vi "Set_Tunnel_Speed_server.vi"(3 "Tunnel Velocity m/s":dbl min=0.0 max=50.0 format="%.2f", 4 "Rig Name":string, 5 "Mode":T1, 6 "Client Name":string="G3_3 HD") -> (0 "Error String":string, 1 "Settling Time (s)":dbl format="%.2f", 2 "Valid Client":bool)   [LabVIEW 2010]
uses:
  ADAM Client/Sub VIs/ADAM Controls/Tunnel_speed_mode.ctl
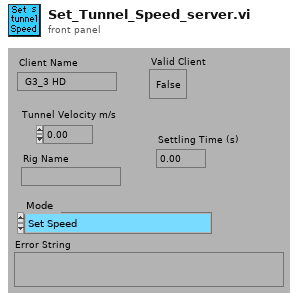
[diagram p1: front panel]
types:
  T1 = typedef "Tunnel_speed_mode.ctl" = enum16{"Set Speed", "Set Speed then wait", "Is tunnel speed allowable?"}
  T2 = typedef "Ch_description_ADAM.ctl" = cluster{"Ch Name":string, "Type":T3, "Function":T4, "Ch State":T5, "Calibration type":T6, "A":dbl, "B":dbl, "C":dbl, "D":dbl, "Comments":string, "Address":T7, "String":string, "Duty":u16}
  T3 = typedef "Module_type_ADAM.ctl" = enum16{"4011", "4012", "4013", "4014", "4016", "4017", "4018", "4021", "4050", "4052", "4053", "4060", "4080", "5000", "5017", "5018", "5024", "5051", "5056", "5060", "6060", "Tracker", "WEST", "GILL", "JEM", "VICI", "Vaisala", "DRUCK", "Run VI Named:", "IR2100", "PPT", "Comparator", "VIRTUAL", "Hold Value", "Read A", "Read Ch", "Coded", "Client Info", "Web Client", "X10", "Test"}
  T4 = typedef "Function_ADAM.ctl" = enum16{"Analogue Input", "Digital Input", "Event counter", "Event rate", "Analogue Output", "Digital Output", "Relay Output"}
  T5 = typedef "Channel_State.ctl" = enum16{"On", "Off", "Always On", "Always Off"}
  T6 = typedef "Calib_type_ADAM.ctl" = enum16{"Raw", "Bx + A", "Cx^2 + Bx + A", "Dx^3 + Cx^2 + Bx + A", "In Band", "Hi-Tec Q", "Hi-Tec M_dot", "Text"}
  T7 = typedef "Address.ctl" = cluster{"Main":i32, "Ch.":i32, "Sub":i32, "Port Name":string}
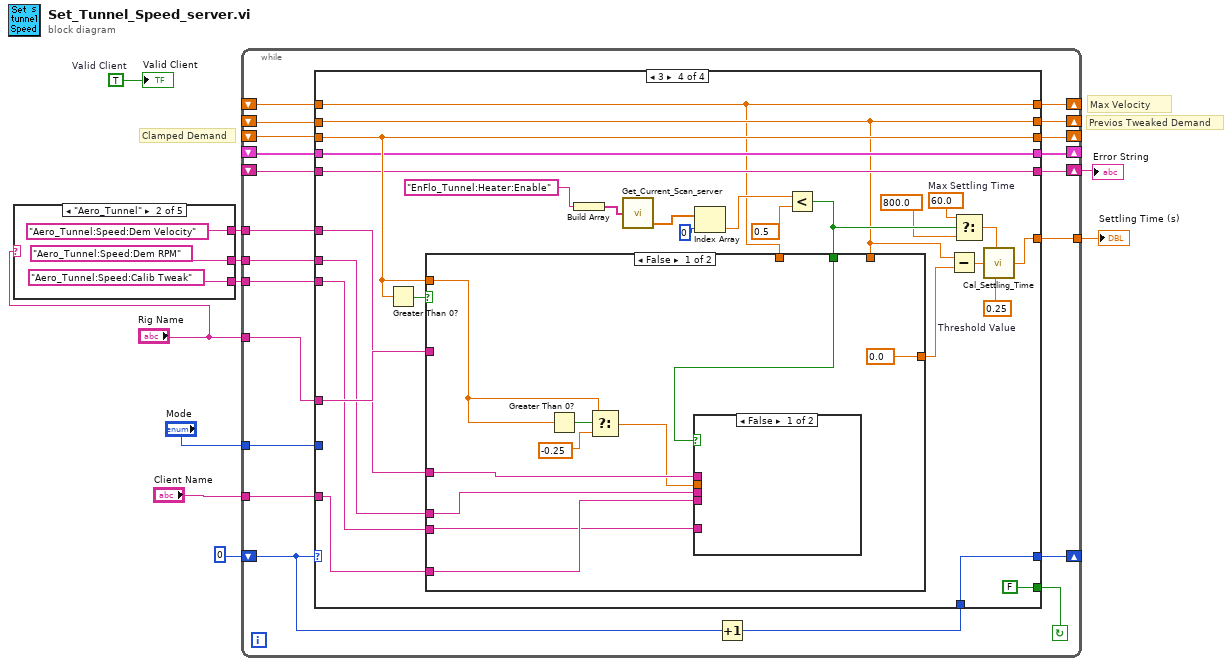
[diagram p0: block diagram]
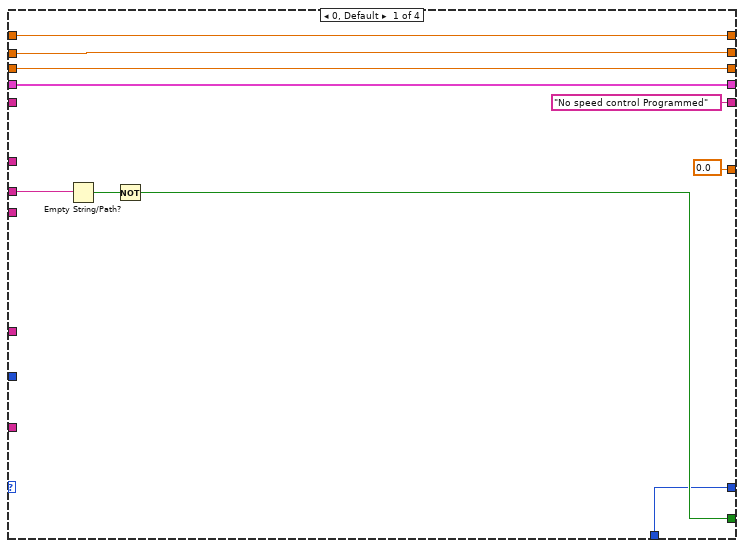
[diagram p2: hidden frame]
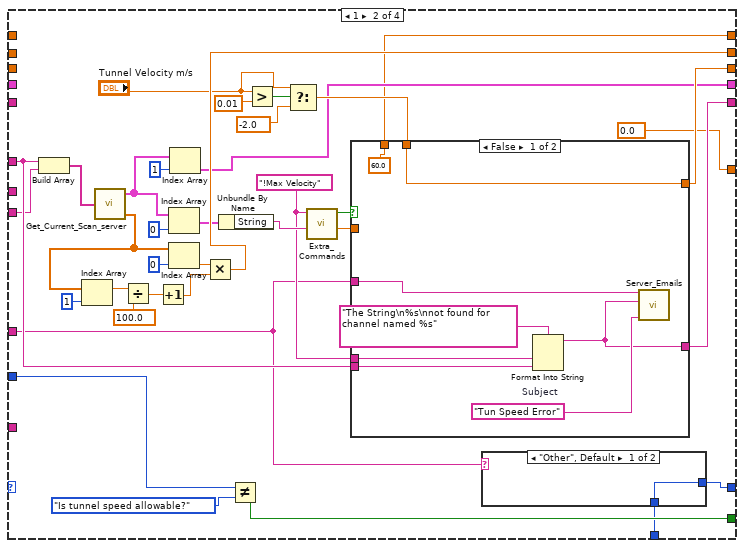
[diagram p3: hidden frame]
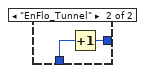
[diagram p4: hidden frame]
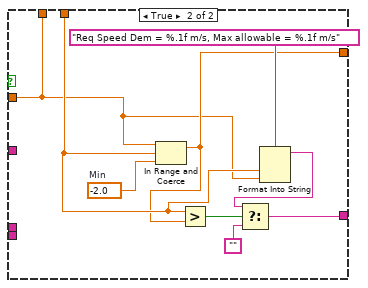
[diagram p5: hidden frame]
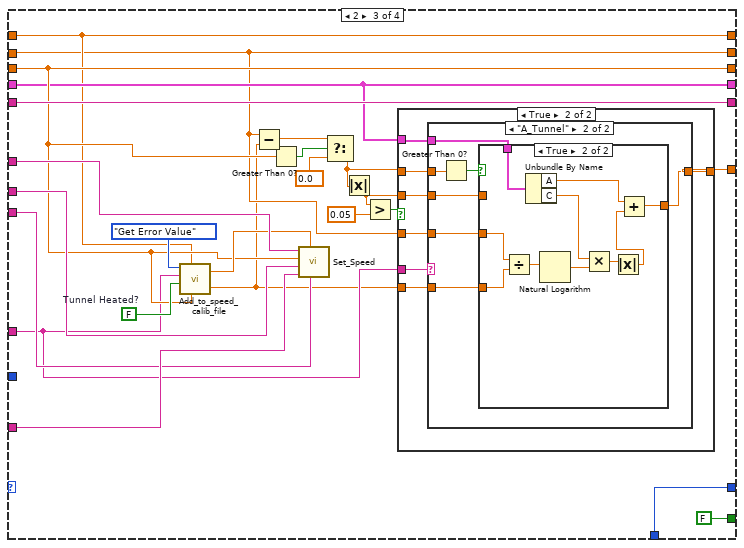
[diagram p6: hidden frame]
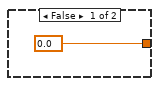
[diagram p7: hidden frame]
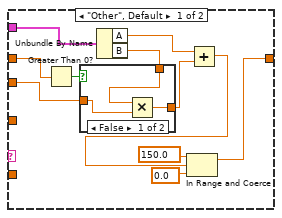
[diagram p8: hidden frame]
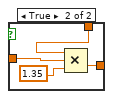
[diagram p9: hidden frame]
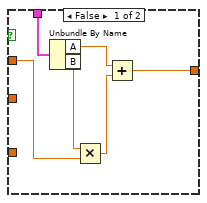
[diagram p10: hidden frame]
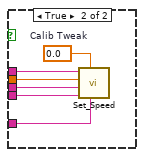
[diagram p11: hidden frame]
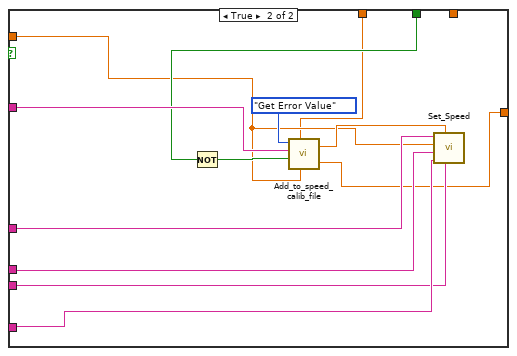
[diagram p12: hidden frame]
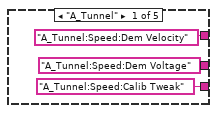
[diagram p13: hidden frame]
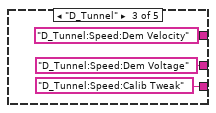
[diagram p14: hidden frame]
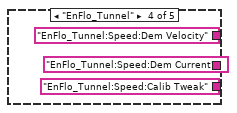
[diagram p15: hidden frame]
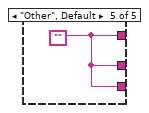
[diagram p16: hidden frame]
diagram:
  w10 = TRUE  # Valid Client
  # "Max Velocity"
  # "Previos Tweaked Demand"
  # "Clamped Demand"
  n1 = case shown="\"Aero_Tunnel\"" "Rig Name" {
    tunnel: ["A_Tunnel:Speed:Dem Velocity" "Aero_Tunnel:Speed:Dem Velocity" "D_Tunnel:Speed:Dem Velocity" "EnFlo_Tunnel:Speed:Dem Velocity" w23] -> w6
    tunnel: ["A_Tunnel:Speed:Dem Voltage" "Aero_Tunnel:Speed:Dem RPM" "D_Tunnel:Speed:Dem Voltage" "EnFlo_Tunnel:Speed:Dem Current" w23] -> w3
    tunnel: ["A_Tunnel:Speed:Calib Tweak" "Aero_Tunnel:Speed:Calib Tweak" "D_Tunnel:Speed:Calib Tweak" "EnFlo_Tunnel:Speed:Calib Tweak" w23] -> w1
    frame "A_Tunnel" {
    }
    frame "Aero_Tunnel" {
    }
    frame "D_Tunnel" {
    }
    frame "EnFlo_Tunnel" {
    }
    frame "Other", Default {
      w23 = ""
    }
  }
  n2 = while {
    shift-left: _ -> [w26]
    shift-right: [w27] -> _
    tunnel: w1 -> [w28]
    shift-left: _ -> [w30]
    shift-right: [w29] -> _
    tunnel: [w31] -> w2
    tunnel: w3 -> [w33]
    shift-left: _ -> [w32]
    shift-right: [w36] -> w5
    shift-left: _ -> [w34]
    shift-right: [w37] -> _
    tunnel: w6 -> [w38]
    shift-left: 0 -> [w41]
    shift-right: [w40] -> _
    tunnel: "Client Name" -> [w43]
    tunnel: "Mode" -> [w44]
    tunnel: "Rig Name" -> [w42]
    shift-right: [w25] -> _
    shift-left: _ -> [w24]
    stop <- w35 continue-if-true
    n3 = Increment(x=w41) -> (x+1=w39:i32)
    n4 = case shown="3" w41 {
      tunnel: w34 -> [w50 _ w122 w199]
      tunnel: w44 -> [_ w80 _ _]
      tunnel: ["No speed control Programmed" w82 w129 w195] -> w36
      tunnel: w43 -> [_ _ w134 w209]
      tunnel: w42 -> [_ w71 w113 w208]
      tunnel: [w51 w74 w132 w200] -> w40
      tunnel: w39 -> [w51 w75 w132 w200]
      tunnel: w38 -> [_ w85 w131 w203]
      tunnel: [w50 w83 w122 w199] -> w37
      tunnel: [w52 w79 FALSE FALSE] -> w35
      tunnel: w33 -> [w54 _ w130 w202]
      tunnel: w32 -> [_ _ w129 w195]
      tunnel: [0.0 ("Settling Time") 0.0 ("Settling Time") w119 w197] -> w31
      tunnel: w30 -> [w48 _ w112 w187]
      tunnel: [w48 w62 w112 w187] -> w29
      tunnel: w28 -> [_ w70 w124 w190]
      tunnel: [w46 w56 w118 w188] -> w27
      tunnel: w26 -> [w46 _ w118 w188]
      tunnel: [w45 w55 w115 w184] -> w25
      tunnel: w24 -> [w45 _ w115 w184]
      frame 0, Default {
        n5 = Empty String/Path?(string/path=w54) -> (empty?=w53:bool)
        n6 = Not(x=w53) -> (.not. x?=w52:bool)
      }
      frame 1 {
        w86 = "!Max Velocity" ("Command")
        n7 = Build Array(w85, w70) -> (w90:string[])
        n8 = call "Get_Current_Scan_server.vi"("Desired Channels"=w90) -> ("Ch Description Array"=w57:T2[], "Numerical Values"=w68:dbl[])  [unwired: 1 out]
        n9 = Index Array(array=w68, index=1 ("Index")) -> (element=w67:dbl)
        n10 = Divide(x=w67, y=100.0) -> (x/y=w65:dbl)
        n11 = Increment(x=w65) -> (x+1=w63:dbl)
        n12 = Index Array(array=w57, index=0 ("Index")) -> (element=w59:T2)
        n13 = Index Array(array=w68, index=0 ("Index")) -> (element=w64:dbl)
        n14 = Index Array(array=w57, index=1 ("Index")) -> (element=w56:T2)
        n15 = Multiply(x=w64, y=w63) -> (x*y=w62:dbl)
        n16 = Unbundle By Name(w59) -> ("String"=w88:string)
        n17 = Not Equal?(x=w80, y=Tunnel_speed_mode."Is tunnel speed allowable?" ("Mode")) -> (x != y?=w79:bool)
        n18 = Greater?(x="Tunnel Velocity m/s", y=0.01) -> (0:w78:bool)
        n19 = Select(t="Tunnel Velocity m/s", s=w78, f=-2.0 ("t")) -> (s? t:f=w76:dbl)
        n20 = call "Extra_Commands.vi"("String to Search"=w88, "Command"=w86) -> ("Numeric Value"=w84:dbl, "Command Found"=w87:bool)  [unwired: 1 in, 3 out]
        n21 = case shown="False" w87 {
          tunnel: w71 -> [w95 _]
          tunnel: w86 -> [w100 _]
          tunnel: w85 -> [w99 _]
          tunnel: w84 -> [_ w102]
          tunnel: w76 -> [w97 w104]
          tunnel: [w97 w103] -> w83
          tunnel: [w96 w106] -> w82
          tunnel: [60.0 ("Numeric Value") w102] -> w55
          frame False {
            w101 = "Tun Speed Error"  # Subject
            n22 = Format Into String(format string="The String\n%s\nnot found for channel named %s" ("Format String"), w100, w99) -> (resulting string=w96:string)  [unwired: 2 in, 1 out]
            n23 = call "Server_Emails.vi"("Client Name Contains"=w95, "Message"=w96, "Subject"=w101) -> ()  [unwired: 2 in, 3 out]
          }
          frame True {
            w110 = -2.0  # Min
            n24 = In Range and Coerce(upper limit=w102, x=w104, lower limit=w110) -> (coerced(x)=w103:dbl)  [unwired: 1 out]
            n25 = Greater?(x=w104, y=w103) -> (0:w105:bool)
            n26 = Format Into String(format string="Req Speed Dem = %.1f m/s, Max allowable = %.1f m/s", w104, w102) -> (resulting string=w108:string)  [unwired: 2 in, 1 out]
            n27 = Select(t=w108, s=w105, f="") -> (s? t:f=w106:string)
          }
        }
        n28 = case shown="\"Other\", Default" w71 {
          tunnel: w75 -> [w91 w93]
          tunnel: [w91 w92] -> w74
          frame "Other", Default {
          }
          frame "EnFlo_Tunnel" {
            n29 = Increment(x=w93) -> (x+1=w92:i32)
          }
        }
      }
      frame 2 {
        w125 = FALSE  # Tunnel Heated?
        n30 = call "Add_to_speed_calib_file.vi"("Desired Velocity"=w122, "Max Velocity"=w115, "Tunnel Heated?"=w125, "Rig Name"=w113, "Mode"=enum16{"Add Row", "Get Error Value"}."Get Error Value") -> ("Tweaked Demand"=w111:dbl, "Calib Tweak %"=w123:dbl)  [unwired: 1 in]
        n31 = Subtract(x=w112, y=w111) -> (x-y=w127:dbl)
        n32 = Greater Than 0?(x=w122) -> (x > 0?=w114:bool)
        n33 = call "Set_Speed.vi"("Channel Name (Calib Tweak)"=w124, "Calib Tweak"=w123, "Client Name"=w134, "Channel Name (Volts/Amps)"=w130, "Demanded Velocity"=w122, "Channel Name (Velocity)"=w131) -> ()  [unwired: 1 in, 4 out]
        n34 = Select(t=w127, s=w114, f=0.0) -> (s? t:f=w117:dbl)
        n35 = Absolute Value(x=w117) -> (abs(x)=w116:dbl)
        n36 = Greater?(x=w116, y=0.05) -> (0:w120:bool)
        n37 = case shown="True" w120 {
          tunnel: w118 -> [_ w142]
          tunnel: [0.0 w139] -> w119
          tunnel: w117 -> [_ w141]
          tunnel: w116 -> [_ w140]
          tunnel: w113 -> [_ w138]
          tunnel: w112 -> [_ w137]
          tunnel: w111 -> [_ w136]
          frame False {
          }
          frame True {
            n38 = case shown="\"A_Tunnel\"" w138 {
              tunnel: w142 -> [w153 w164]
              tunnel: w141 -> [w148 w166]
              tunnel: w140 -> [w144 w165]
              tunnel: [w143 w163] -> w139
              tunnel: w137 -> [_ w162]
              tunnel: w136 -> [_ w161]
              frame "Other", Default {
                n39 = Greater Than 0?(x=w148) -> (x > 0?=w147:bool)
                n40 = Unbundle By Name(w153) -> ("A"=w152:dbl, "B"=w146:dbl)
                n41 = case shown="False" w147 {
                  tunnel: [w156 w157] -> w145
                  tunnel: w146 -> [w155 w160]
                  tunnel: w144 -> [w154 w159]
                  frame False {
                    n42 = Multiply(x=w155, y=w154) -> (x*y=w156:dbl)
                  }
                  frame True {
                    n43 = Compound Arithmetic op=MULTIPLY(w160, w159, 1.35 ("Min")) -> (w157:dbl)
                  }
                }
                n44 = Add(x=w152, y=w145) -> (x+y=w149:dbl)
                n45 = In Range and Coerce(upper limit=150.0 ("Max"), x=w149, lower limit=0.0 ("Min")) -> (coerced(x)=w143:dbl)  [unwired: 1 out]
              }
              frame "A_Tunnel" {
                n46 = Greater Than 0?(x=w166) -> (x > 0?=w167:bool)
                n47 = case shown="True" w167 {
                  tunnel: w165 -> [w169 _]
                  tunnel: w164 -> [w173 w183]
                  tunnel: [w168 w174] -> w163
                  tunnel: w162 -> [_ w181]
                  tunnel: w161 -> [_ w180]
                  frame False {
                    n48 = Unbundle By Name(w173) -> ("A"=w172:dbl, "B"=w170:dbl)
                    n49 = Multiply(x=w170, y=w169) -> (x*y=w171:dbl)
                    n50 = Add(x=w172, y=w171) -> (x+y=w168:dbl)
                  }
                  frame True {
                    n51 = Divide(x=w181, y=w180) -> (x/y=w182:dbl)
                    n52 = Unbundle By Name(w183) -> ("A"=w175:dbl, "C"=w178:dbl)
                    n53 = Natural Logarithm(1:w182) -> (0:w179:dbl)
                    n54 = Multiply(x=w178, y=w179) -> (x*y=w177:dbl)
                    n55 = Absolute Value(x=w177) -> (abs(x)=w176:dbl)
                    n56 = Add(x=w175, y=w176) -> (x+y=w174:dbl)
                  }
                }
              }
            }
          }
        }
      }
      frame 3 {
        w198 = 0.25  # Threshold Value
        w193 = 60.0  # Max Settling Time
        n57 = Greater Than 0?(x=w199) -> (x > 0?=w210:bool)
        n58 = Build Array("EnFlo_Tunnel:Heater:Enable") -> (w186:string[])
        n59 = call "Get_Current_Scan_server.vi"("Desired Channels"=w186) -> ("Numerical Values"=w185:dbl[])  [unwired: 2 out]
        n60 = Index Array(array=w185, index=0) -> (element=w204:dbl)
        n61 = Less?(x=w204, y=0.5) -> (x < y?=w194:bool)
        n62 = case shown="False" w210 {
          tunnel: w199 -> [w218 w228]
          tunnel: w203 -> [w217 w238]
          tunnel: w202 -> [w215 w237]
          tunnel: w209 -> [w214 w236]
          tunnel: w208 -> [_ w235]
          tunnel: w194 -> [w213 w233]
          tunnel: [0.0 w229] -> w189
          tunnel: w190 -> [w211 w231]
          tunnel: w187 -> [_ _]
          tunnel: w184 -> [_ w227]
          frame False {
            n63 = Greater Than 0?(x=w218) -> (x > 0?=w220:bool)
            n64 = Select(t=w218, s=w220, f=-0.25 ("t")) -> (s? t:f=w216:dbl)
            n65 = case shown="False" w213 {
              tunnel: w217 -> [_ w226]
              tunnel: w216 -> [_ w225]
              tunnel: w215 -> [_ w224]
              tunnel: w214 -> [_ w223]
              tunnel: w211 -> [_ w222]
              frame False {
              }
              frame True {
                w221 = 0.0  # Calib Tweak
                n66 = call "Set_Speed.vi"("Channel Name (Calib Tweak)"=w222, "Calib Tweak"=w221, "Client Name"=w223, "Channel Name (Volts/Amps)"=w224, "Demanded Velocity"=w225, "Channel Name (Velocity)"=w226) -> ()  [unwired: 1 in, 4 out]
              }
            }
          }
          frame True {
            n67 = Not(x=w233) -> (.not. x?=w232:bool)
            n68 = call "Add_to_speed_calib_file.vi"("Desired Velocity"=w228, "Max Velocity"=w227, "Tunnel Heated?"=w232, "Rig Name"=w235, "Mode"=enum16{"Add Row", "Get Error Value"}."Get Error Value") -> ("Tweaked Demand"=w229:dbl, "Calib Tweak %"=w230:dbl)  [unwired: 1 in]
            n69 = call "Set_Speed.vi"("Channel Name (Calib Tweak)"=w231, "Calib Tweak"=w230, "Client Name"=w236, "Channel Name (Volts/Amps)"=w237, "Demanded Velocity"=w228, "Channel Name (Velocity)"=w238) -> ()  [unwired: 1 in, 4 out]
          }
        }
        n70 = Subtract(x=w187, y=w189) -> (x-y=w196:dbl)
        n71 = Select(t=w193, s=w194, f=800.0) -> (s? t:f=w191:dbl)
        n72 = call "Cal_Settling_Time.vi"("Max Settling Time"=w191, "Speed Tweak (m/s)"=w196, "Threshold Value"=w198) -> ("Required Settling Time"=w197:dbl)  [unwired: 2 out]
      }
    }
  }
  "Error String" <- w5
  "Settling Time (s)" <- w2
  "Valid Client" <- w10
